vi "Set Item Property (Dependent File).vi"(6 "OptionalInfo":T1, 8 "error in (no error)":errorcluster, 9 "Path":path, 10 "Property Name":string, 11 "Item Ref in":T2 format="%.0x") -> (0 "error out":errorcluster, 3 "Item Ref out":T2 format="%.0x", 4 "Replaced":bool)   [LabVIEW 2026, in "Custom Devices Storage.lvlib"]
uses:
  Custom Devices Storage.lvlib
  <vilib>/NI VeriStand/Custom Device API/Custom Device Item Ref.ctl
  <vilib>/NI VeriStand/Custom Device API/Custom Device API.lvlib
  <vilib>/NI VeriStand/Custom Device API/Dependent File Optional Info.ctl
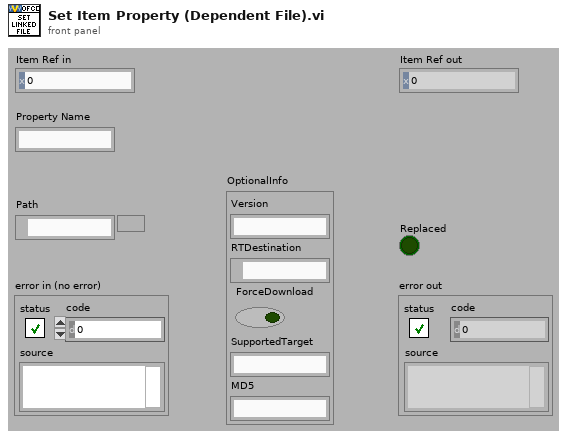
[diagram p1: front panel]
types:
  T1 = typedef "Custom Device API.lvlib/Dependent File Optional Info.ctl" = cluster{"Version":string, "RTDestination":path, "ForceDownload":bool, "SupportedTarget":string, "MD5":string}
  T2 = typedef "Custom Device API.lvlib/Custom Device Item Ref.ctl" = u64
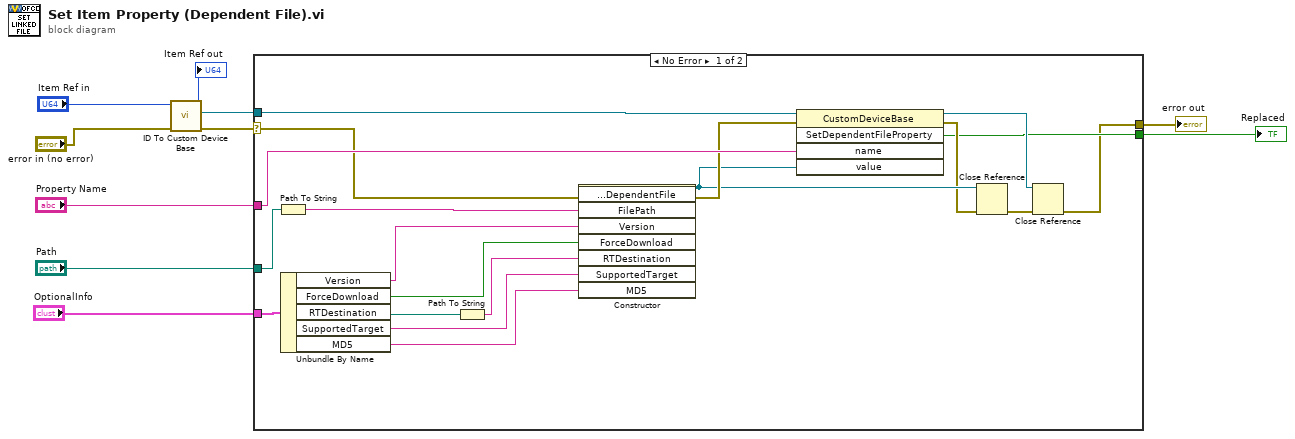
[diagram p0: block diagram]
diagram:
  n1 = call "ID To Custom Device Base.vi"("error in (no error)"="error in (no error)", "ID in"="Item Ref in") -> ("error out"=w7:errorcluster, "BaseNode"=w6:refnum<k39>, "ID out"=→"Item Ref out":u64)  [unwired: 7 in]
  n2 = case shown="No Error" w7 {
    selector: w7 -> [w27 w30]
    tunnel: w6 -> [w29 _]
    tunnel: "Property Name" -> [w28 _]
    tunnel: "OptionalInfo" -> [w17 _]
    tunnel: "Path" -> [w25 _]
    tunnel: [w19 _] -> w2
    tunnel: [w18 w30] -> w1
    frame No Error {
      n3 = Path To String(path=w25) -> (string=w24:string)
      n4 = Unbundle By Name(w17) -> ("Version"=w15:string, "ForceDownload"=w14:bool, "RTDestination"=w16:path, "SupportedTarget"=w12:string, "MD5"=w11:string)
      n5 = Path To String(path=w16) -> (string=w13:string)
      n6 = constructor class="DependentFile"(error in=w27, "FilePath"=w24, "Version"=w15, "ForceDownload"=w14, "RTDestination"=w13, "SupportedTarget"=w12, "MD5"=w11) -> (reference out=w23:refnum<k39>, error out=w26:errorcluster)  [unwired: 2 in, 7 out]
      n7 = invoke class="CustomDeviceBase" method="SetDependentFileProperty"(reference=w29, error in=w26, "name"=w28, "value"=w23) -> (reference out=w20:refnum<k39>, error out=w22:errorcluster, "SetDependentFileProperty"=w19:bool)  [unwired: 1 in, 2 out]
      n8 = Close Reference(reference=w23, error in (no error)=w22) -> (error out=w21:errorcluster)
      n9 = Close Reference(reference=w20, error in (no error)=w21) -> (error out=w18:errorcluster)
    }
    frame Error {
    }
  }
  "error out" <- w1
  "Replaced" <- w2
